vi "ACT_Loop.vi"() -> ()   [LabVIEW 2020, in "Arm_ACT.lvlib"]
uses:
  Arm_ACT.lvlib
  Cluster_CMD_ACT_Data.ctl
  ENUM_ACT_State.ctl
  Type Defs/Talon_FX_Control_Module.ctl
  <vilib>/Rock Robotics/WPI/MotorControl/WPI_MotorControlDeviceRef.ctl
  <vilib>/Rock Robotics/WPI/MotorControl/WPI_MotorControlType.ctl
  <vilib>/Rock Robotics/SystemInterfaces/DIO/FPGA_DIOPWMChannel.ctl
  <vilib>/Rock Robotics/WPI/PWM/WPI_PWMDeadband.ctl
  <vilib>/Rock Robotics/SystemInterfaces/DIO/FPGA_DIOChannel.ctl
  <vilib>/Rock Robotics/WPI/ThirdParty/Phoenix-LabVIEW/Motor Controller/Controls/CTRE_Phoenix_MotorControl_ControlMode.ctl
  ENUM_ACT_Action.ctl
  Utility/Global_STOP.vi
  Global_CMD_ACT_Data In.vi
  <vilib>/Rock Robotics/WPI/ThirdParty/Phoenix-LabVIEW/Motor Controller/Get/CTRE_Phoenix_MotorController_GetLimitSwitchStates.vi
  <vilib>/Rock Robotics/WPI/ThirdParty/Phoenix-LabVIEW/Motor Controller/Get/CTRE_Phoenix_MotorController_GetSelectedSensorData.vi
  Global_ACT_Data Out.vi
panel:
  in  "Arm Offset (Inches)":dbl
  in  "Wrist Offset (Inches)":dbl
  in  "Using Inverse Kinematics?":bool
  in  "arm angle":dbl(slide) scale=0.0..1.0
  out "Input DBL Data":T1
  out "Output DBL Data":dbl
  out "Cycle Time (S)":dbl format="%.3g"
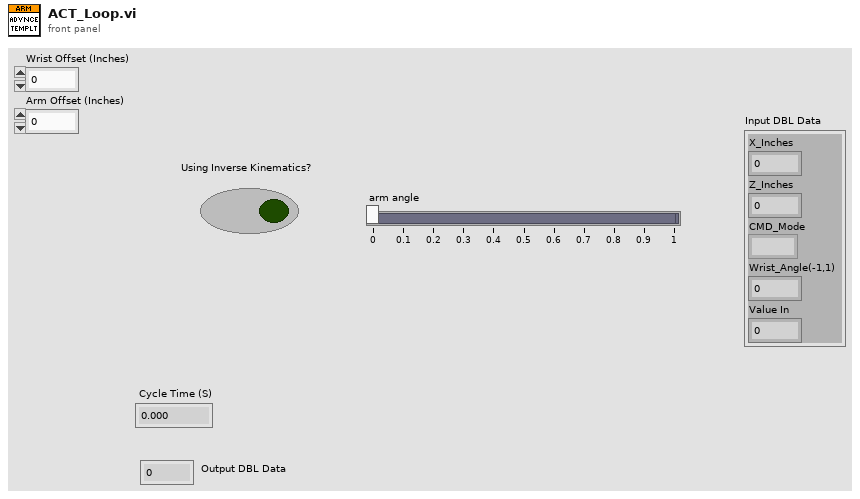
[diagram p1: front panel]
types:
  T1 = typedef "Arm_ACT.lvlib/Cluster_CMD_ACT_Data.ctl" = cluster{"X_Inches":dbl, "Z_Inches":dbl, "CMD_Mode":enum16{""}, "Wrist_Angle(-1,1)":dbl, "Value In":dbl}
  T2 = typedef "Talon_FX_Control_Module.ctl" = cluster{"MotorDevRef":T3, "Control Mode":T8, "Output":dbl}
  T3 = typedef "WPI_MotorControlDeviceRef.ctl" = cluster{"DeviceStatus":errorcluster, "Type":T4, "PWM":cluster{"PWM Channel":T5, "DeadBand":T6}, "CAN":cluster{"Device Number":u8, "SetOutput VI Ref":variant, "GetOutput VI Ref":variant, "Enable VI Ref":variant, "Disable VI Ref":variant, "Data":variant}, "Invert":bool, "DIO PWM":cluster{"PWM \"Enable\" Channel":T5, "DIOChannel":T7, "PWM Rate":dbl}}
  T4 = typedef "WPI_MotorControlType.ctl" = enum16{"PWM", "CAN", "DIO PWM"}
  T5 = typedef "FPGA_DIOPWMChannel.ctl" = enum8{"PWM 0", "PWM 1", "PWM 2", "PWM 3", "PWM 4", "PWM 5", "PWM 6", "PWM 7", "PWM 8", "PWM 9", "PWM MXP 0", "PWM MXP 1", "PWM MXP 2", "PWM MXP 3", "PWM MXP 4", "PWM MXP 5", "PWM MXP 6", "PWM MXP 7", "PWM MXP 8", "PWM MXP 9", "Invalid"}
  T6 = typedef "WPI_PWMDeadband.ctl" = cluster{"Name":string, "maxPositivePwm":i32, "minPositivePwm":i32, "centerPwm":i32, "maxNegativePwm":i32, "minNegativePwm":i32, "angularRange":u16}
  T7 = typedef "FPGA_DIOChannel.ctl" = enum8{"DIO 0", "DIO 1", "DIO 2", "DIO 3", "DIO 4", "DIO 5", "DIO 6", "DIO 7", "DIO 8", "DIO 9", "DIO MXP 0", "DIO MXP 1", "DIO MXP 2", "DIO MXP 3", "DIO MXP 4", "DIO MXP 5", "DIO MXP 6", "DIO MXP 7", "DIO MXP 8", "DIO MXP 9", "DIO MXP 10", "DIO MXP 11", "DIO MXP 12", "DIO MXP 13", "DIO MXP 14", "DIO MXP 15", "SPI Port CS1", "SPI Port CS2", "SPI Port CS3", "SPI Port MISO", "SPI Port MOSI", "Invalid"}
  T8 = typedef "CTRE_Phoenix_MotorControl_ControlMode.ctl" = u16
  T9 = typedef "Arm_ACT.lvlib/ENUM_ACT_State.ctl" = enum16{"Startup", "Set Motors", "Inverse Kinematics Set Motors", "Shutdown"}
  T10 = cluster{"Wrist CM":T2, "Shoulder CM":T2, "Extender CM":T2, "State":T9, "Previous State":T9, "Current Time":timestamp, "Previous Time":timestamp, "Start Time":timestamp, "Target Time (ms)":u32, "Cycle Time(S)":dbl, "ACT Input":T1, "ACT Output DBL":dbl}
  T11 = typedef "Arm_ACT.lvlib/ENUM_ACT_Action.ctl" = enum16{"No Action", "Reset Time", "Reset All", "Zero Motors", "Config Motors", "Set Arm Position", "Set Motors Inverse Kinematics", "Set Wrist Angle"}
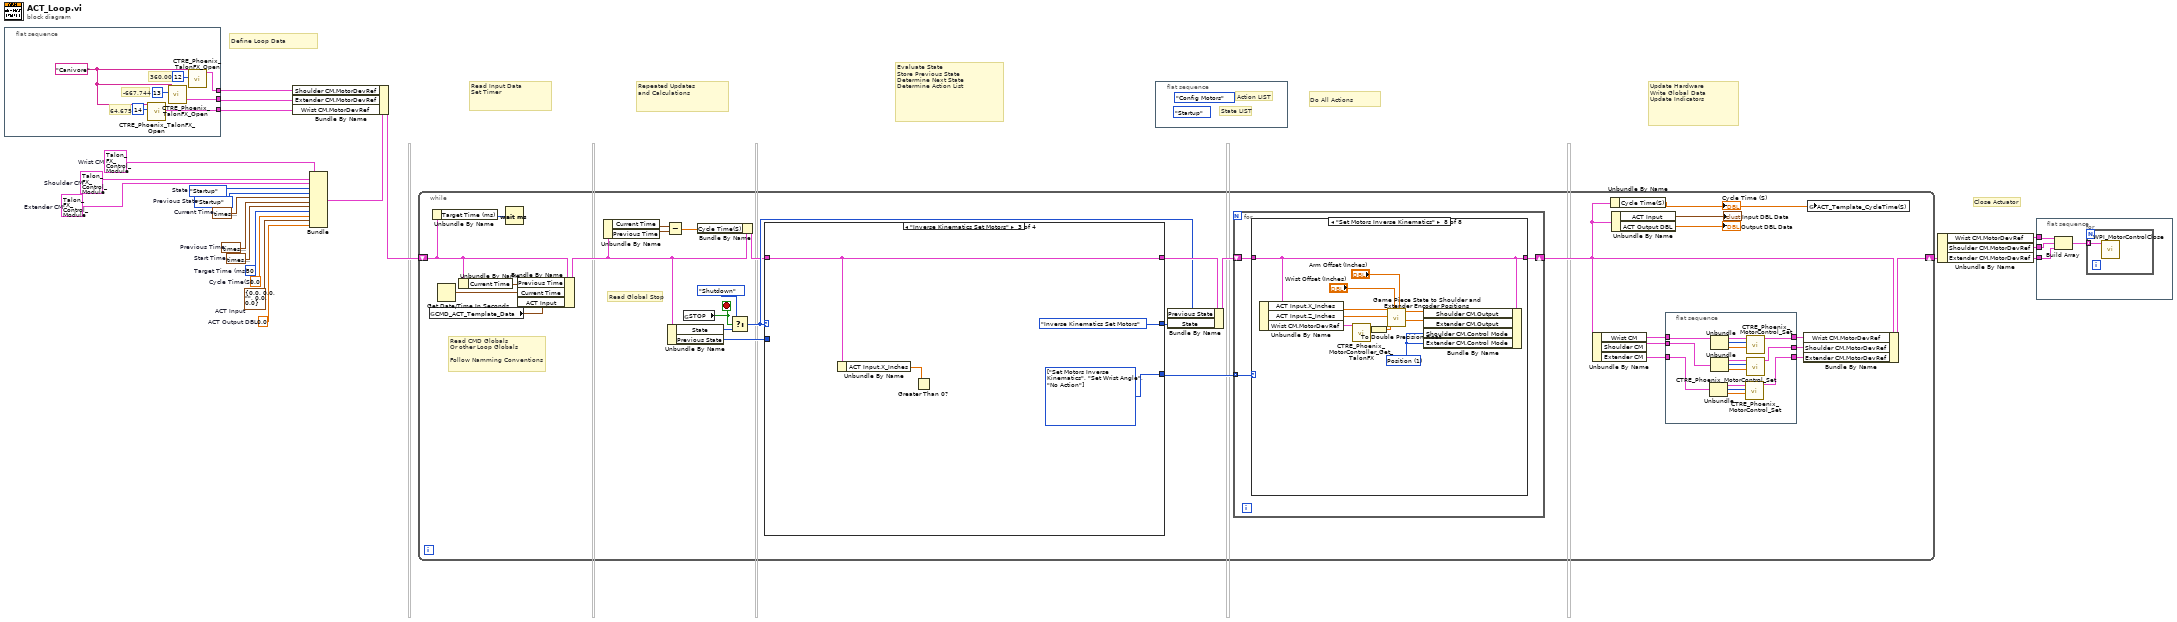
[diagram p0: block diagram]
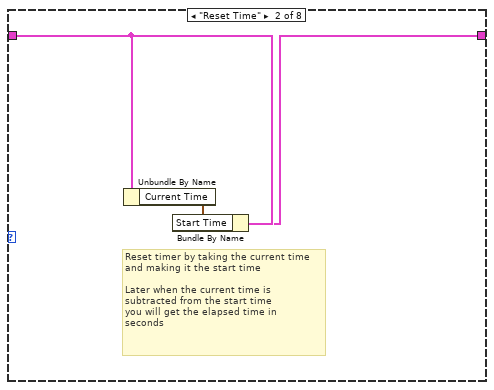
[diagram p3: hidden frame]
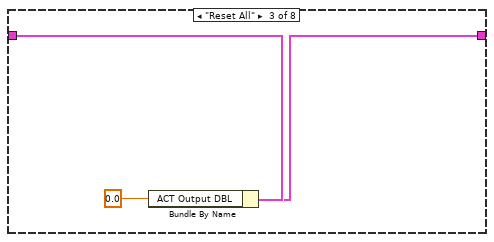
[diagram p4: hidden frame]
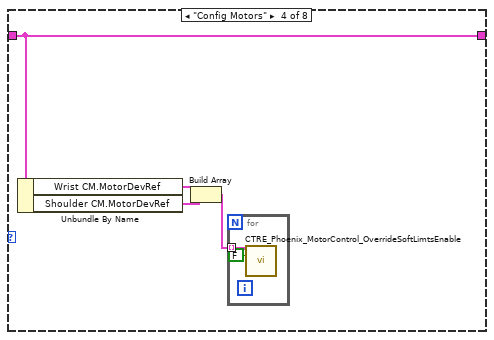
[diagram p5: hidden frame]
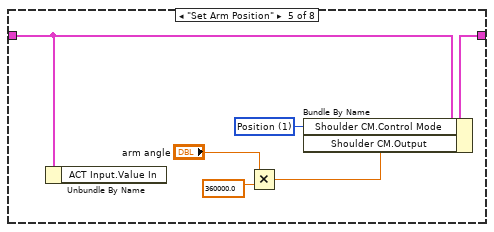
[diagram p6: hidden frame]
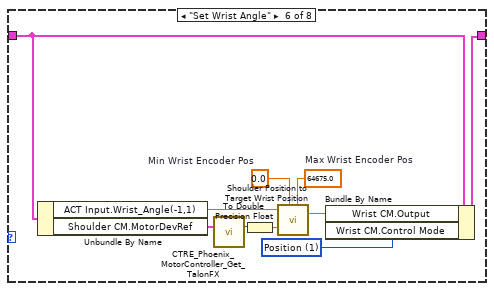
[diagram p7: hidden frame]
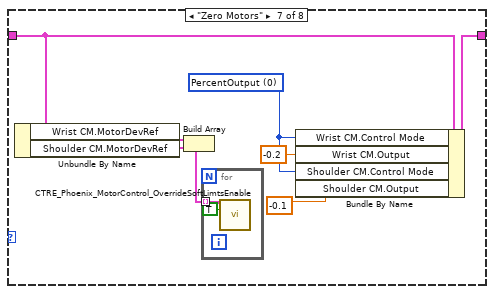
[diagram p8: hidden frame]
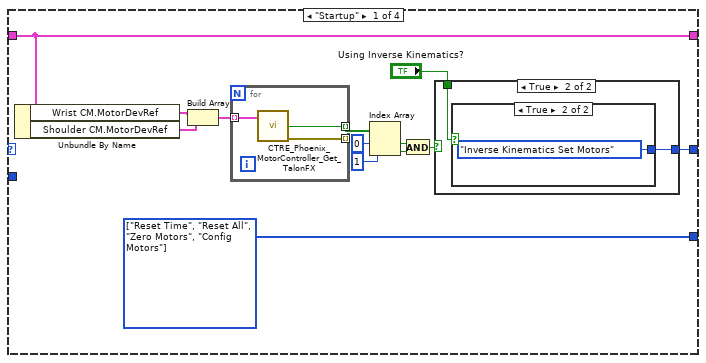
[diagram p9: hidden frame]
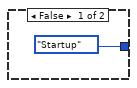
[diagram p10: hidden frame]
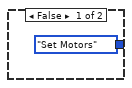
[diagram p11: hidden frame]
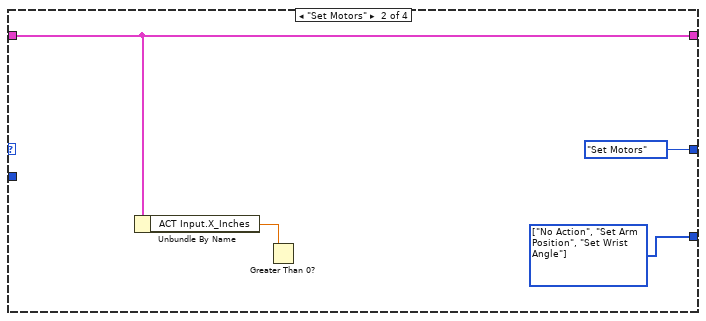
[diagram p12: hidden frame]
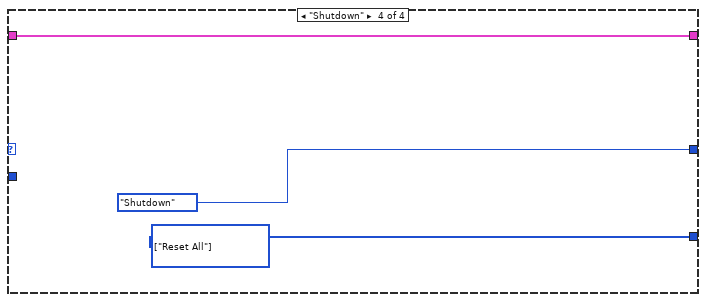
[diagram p13: hidden frame]
diagram:
  w1 = T2 {"MotorDevRef"={"DeviceStatus"={"status"=FALSE, "code"=0, "source"=""}, "Type"=enum."PWM", "PWM"={"PWM Channel"=enum."PWM 1", "DeadBand"={"Name"="", "maxPositivePwm"=0, "minPositivePwm"=0, "centerPwm"=0, "maxNegativePwm"=0, "minNegativePwm"=0, "angularRange"=0}}, "CAN"={"Device Number"=0, "SetOutput VI Ref"=variant(enum8{"Percent VBus", "Current", "Speed", "Position", "Voltage"} enum."Percent VBus"), "GetOutput VI Ref"=variant(refnum<k1> refnum), "Enable VI Ref"=variant(dbl 12.0), "Disable VI Ref"=variant(enum8{"Percent VBus", "Speed", "Position", "Slave", "Unchanged / Invalid", "Voltage Compensation", "Current", "Motion Profile"} enum."Percent VBus"), "Data"=variant}, "Invert"=FALSE, "DIO PWM"={"PWM \"Enable\" Channel"=enum."Invalid", "DIOChannel"=enum."Invalid", "PWM Rate"=0.0}}, "Control Mode"=0, "Output"=0.0}  # Extender CM
  w2 = T2 {"MotorDevRef"={"DeviceStatus"={"status"=FALSE, "code"=0, "source"=""}, "Type"=enum."PWM", "PWM"={"PWM Channel"=enum."PWM 1", "DeadBand"={"Name"="", "maxPositivePwm"=0, "minPositivePwm"=0, "centerPwm"=0, "maxNegativePwm"=0, "minNegativePwm"=0, "angularRange"=0}}, "CAN"={"Device Number"=0, "SetOutput VI Ref"=variant(enum8{"Percent VBus", "Current", "Speed", "Position", "Voltage"} enum."Percent VBus"), "GetOutput VI Ref"=variant(refnum<k1> refnum), "Enable VI Ref"=variant(dbl 12.0), "Disable VI Ref"=variant(enum8{"Percent VBus", "Speed", "Position", "Slave", "Unchanged / Invalid", "Voltage Compensation", "Current", "Motion Profile"} enum."Percent VBus"), "Data"=variant}, "Invert"=FALSE, "DIO PWM"={"PWM \"Enable\" Channel"=enum."Invalid", "DIOChannel"=enum."Invalid", "PWM Rate"=0.0}}, "Control Mode"=0, "Output"=0.0}  # Shoulder CM
  w3 = T2 {"MotorDevRef"={"DeviceStatus"={"status"=FALSE, "code"=0, "source"=""}, "Type"=enum."PWM", "PWM"={"PWM Channel"=enum."PWM 1", "DeadBand"={"Name"="", "maxPositivePwm"=0, "minPositivePwm"=0, "centerPwm"=0, "maxNegativePwm"=0, "minNegativePwm"=0, "angularRange"=0}}, "CAN"={"Device Number"=0, "SetOutput VI Ref"=variant(enum8{"Percent VBus", "Current", "Speed", "Position", "Voltage"} enum."Percent VBus"), "GetOutput VI Ref"=variant(refnum<k1> refnum), "Enable VI Ref"=variant(dbl 12.0), "Disable VI Ref"=variant(enum8{"Percent VBus", "Speed", "Position", "Slave", "Unchanged / Invalid", "Voltage Compensation", "Current", "Motion Profile"} enum."Percent VBus"), "Data"=variant}, "Invert"=FALSE, "DIO PWM"={"PWM \"Enable\" Channel"=enum."Invalid", "DIOChannel"=enum."Invalid", "PWM Rate"=0.0}}, "Control Mode"=0, "Output"=0.0}  # Wrist CM
  w13 = 0.0  # Cycle Time(S)
  w14 = ENUM_ACT_State."Startup"  # Previous State
  w15 = timestamp(0 s since 1904-01-01)  # Previous Time
  w16 = u32 50  # Target Time (ms)
  w17 = 0.0  # ACT Output DBL
  w18 = T1 {"X_Inches"=0.0, "Z_Inches"=0.0, "CMD_Mode"=enum."", "Wrist_Angle(-1,1)"=0.0, "Value In"=0.0}  # ACT Input
  w19 = timestamp(0 s since 1904-01-01)  # Start Time
  w20 = timestamp(0 s since 1904-01-01)  # Current Time
  w21 = ENUM_ACT_State."Startup"  # State
  # "Close Actuator"
  # "Define Loop Data"
  # "Repeated Updates\nand Calculations"
  # "Read Input Data\nSet Timer"
  # "Evaluate State\nStore Previous State\nDetermine Next State\nDetermine Action List"
  # "Do All Actions"
  # "Update Hardware\nWrite Global Data\nUpdate Indicators"
  n1 = flat-sequence {
    tunnel: [w27] -> w8
    tunnel: [w25] -> w7
    tunnel: [w23] -> w6
    frame #0 {
      w22 = "Canivore" ("CAN Bus")
      # "360,000"
      # "-667,744"
      # "64,675"
      n2 = call <vilib>:"CTRE_Phoenix_TalonFX_Open.vi"("Device Number"=u8 14, "CAN Bus"=w22) -> ("PhoenixMotorControlDevRef"=w27:T3)  [unwired: 8 in, 1 out]
      n3 = call <vilib>:"CTRE_Phoenix_TalonFX_Open.vi"("Device Number"=u8 13, "CAN Bus"=w22) -> ("PhoenixMotorControlDevRef"=w25:T3)  [unwired: 8 in, 1 out]
      n4 = call <vilib>:"CTRE_Phoenix_TalonFX_Open.vi"("Device Number"=u8 12, "CAN Bus"=w22) -> ("PhoenixMotorControlDevRef"=w23:T3)  [unwired: 8 in, 1 out]
    }
  }
  n5 = Bundle("Wrist CM"=w3, "Shoulder CM"=w2, "Extender CM"=w1, "State"=w21, "Previous State"=w14, "Current Time"=w20, "Previous Time"=w15, "Start Time"=w19, "Target Time (ms)"=w16, "Cycle Time(S)"=w13, "ACT Input"=w18, "ACT Output DBL"=w17) -> (w10:T10)  [unwired: 1 in]
  n6 = Bundle By Name(cluster=w10, "Shoulder CM.MotorDevRef"=w6, "Extender CM.MotorDevRef"=w7, "Wrist CM.MotorDevRef"=w8) -> (w9:T10)
  n7 = while {
    shift-right: [w37] -> w11
    shift-left: w9 -> [w33]
    stop <- w54 stop-if-true
    # "Read CMD Globals\nOr other Loop Globals\n\nFollow Namming Conventions"
    # "Read Global Stop"
    n8 = global read "Global_CMD_ACT_Data In.vi" "CMD_ACT_Template_Data"() -> (w39:T1)
    n9 = Unbundle By Name(w33) -> ("Target Time (ms)"=w51:u32)
    n10 = Get Date/Time In Seconds() -> (seconds since 1Jan1904=w58:timestamp)
    n11 = Unbundle By Name(w33) -> ("Current Time"=w50:timestamp)
    n12 = Wait (ms)(milliseconds to wait=w51) -> ()  [unwired: 1 out]
    n13 = Bundle By Name(cluster=w33, "Previous Time"=w50, "Current Time"=w58, "ACT Input"=w39) -> (w44:T10)
    n14 = Unbundle By Name(w44) -> ("Current Time"=w45:timestamp, "Previous Time"=w46:timestamp)
    n15 = Subtract(x=w45, y=w46) -> (x-y=w42:dbl)
    n16 = Unbundle By Name(w44) -> ("State"=w52:T9, "Previous State"=w49:T9)
    n17 = global read "Global_STOP.vi" "STOP"() -> (w54:bool)
    n18 = Bundle By Name(cluster=w44, "Cycle Time(S)"=w42) -> (w43:T10)
    n19 = Select(t=ENUM_ACT_State."Shutdown" ("State"), s=w54, f=w52) -> (s? t:f=w47:T9)
    n20 = case shown="\"Inverse Kinematics Set Motors\"" w47 {
      tunnel: w43 -> [w137 w149 w153 w158]
      tunnel: [w137 w149 w153 w158] -> w56
      tunnel: [w138 ENUM_ACT_State."Set Motors" ("State") ENUM_ACT_State."Inverse Kinematics Set Motors" ("State") ENUM_ACT_State."Shutdown" ("State")] -> w55
      tunnel: [w139 w148 w152 w156] -> w41
      tunnel: w49 -> [_ _ _ _]
      frame "Startup" {
        w139 = T11[] [enum."Reset Time", enum."Reset All", enum."Zero Motors", enum."Config Motors"] items=["No Action", "Reset Time", "Reset All", "Zero Motors", "Config Motors", "Set Arm Position", "Set Motors Inverse Kinematics", "Set Wrist Angle"] ("Actions")
        n21 = Unbundle By Name(w137) -> ("Wrist CM.MotorDevRef"=w136:T3, "Shoulder CM.MotorDevRef"=w128:T3)
        n22 = Build Array(w136, w128) -> (w134:T3[])
        n23 = for {
          tunnel: w134 -> [w142] mode=indexing
          tunnel: [w141] -> w133 mode=indexing
          tunnel: [w140] -> _ mode=indexing
          n24 = call-poly <vilib>:"CTRE_Phoenix_MotorController_Get_TalonFX.vi"("PhoenixMotorControlDevRef"=w142) -> ("Reverse Limit Closed?"=w141:bool, "error out"=w140:errorcluster)  [unwired: 11 in, 2 out]
        }
        n25 = Index Array(array=w133, index #1=0 ("index"), index #2=1 ("index")) -> (element #1=w130:bool, element #2=w129:bool)
        n26 = And(x=w130, y=w129) -> (x .and. y?=w135:bool)
        n27 = case shown="True" w135 {
          tunnel: [ENUM_ACT_State."Startup" ("State") w145] -> w138
          tunnel: "Using Inverse Kinematics?" -> [_ w144]
          frame False {
          }
          frame True {
            n28 = case shown="True" w144 {
              tunnel: [ENUM_ACT_State."Set Motors" ("State") ENUM_ACT_State."Inverse Kinematics Set Motors" ("State")] -> w145
              frame False {
              }
              frame True {
              }
            }
          }
        }
      }
      frame "Set Motors" {
        w148 = T11[] [enum."No Action", enum."Set Arm Position", enum."Set Wrist Angle"] items=["No Action", "Reset Time", "Reset All", "Zero Motors", "Config Motors", "Set Arm Position", "Set Motors Inverse Kinematics", "Set Wrist Angle"] ("Actions")
        n29 = Unbundle By Name(w149) -> ("ACT Input.X_Inches"=w151:dbl)
        n30 = Greater Than 0?(x=w151) -> ()  [unwired: 1 out]
      }
      frame "Inverse Kinematics Set Motors" {
        w152 = T11[] [enum."Set Motors Inverse Kinematics", enum."Set Wrist Angle", enum."No Action"] items=["No Action", "Reset Time", "Reset All", "Zero Motors", "Config Motors", "Set Arm Position", "Set Motors Inverse Kinematics", "Set Wrist Angle"] ("Actions")
        n31 = Unbundle By Name(w153) -> ("ACT Input.X_Inches"=w155:dbl)
        n32 = Greater Than 0?(x=w155) -> ()  [unwired: 1 out]
      }
      frame "Shutdown" {
        w156 = T11[] [enum."Reset All"] items=["No Action", "Reset Time", "Reset All", "Zero Motors", "Config Motors", "Set Arm Position", "Set Motors Inverse Kinematics", "Set Wrist Angle"] ("Actions")
      }
    }
    n33 = Bundle By Name(cluster=w56, "Previous State"=w47, "State"=w55) -> (w57:T10)
    n34 = for {
      tunnel: w41 -> [w76] mode=indexing
      shift-right: [w75] -> w38
      shift-left: w57 -> [w74]
      n35 = case shown="\"Set Motors Inverse Kinematics\"" w76 {
        tunnel: w74 -> [w77 w80 w83 w85 w95 w99 w110 w119]
        tunnel: [w77 w79 w82 w85 w94 w98 w109 w119] -> w75
        frame "No Action" {
        }
        frame "Reset Time" {
          # "Reset timer by taking the current time\nand making it the start time\n\nLater when the current time is \nsubtracted from the start time\nyou will get the elapsed time in \nseconds"
          n36 = Unbundle By Name(w80) -> ("Current Time"=w78:timestamp)
          n37 = Bundle By Name(cluster=w80, "Start Time"=w78) -> (w79:T10)
        }
        frame "Reset All" {
          n38 = Bundle By Name(cluster=w83, "ACT Output DBL"=0.0 ("FG Write Value")) -> (w82:T10)
        }
        frame "Config Motors" {
          n39 = Unbundle By Name(w85) -> ("Wrist CM.MotorDevRef"=w87:T3, "Shoulder CM.MotorDevRef"=w86:T3)
          n40 = Build Array(w87, w86) -> (w84:T3[])
          n41 = for {
            tunnel: w84 -> [w89] mode=indexing
            n42 = call <vilib>:"CTRE_Phoenix_MotorControl_OverrideSoftLimtsEnable.vi"("PhoenixMotorControlDevRef"=w89, "Override Soft Limit Enable?"=FALSE) -> ()  [unwired: 12 in, 2 out]
          }
        }
        frame "Set Arm Position" {
          w93 = T8 1 items=["PercentOutput"=0, "Position"=1, "Velocity"=2, "Current"=3, "Follower"=5, "MotionProfile"=6, "MotionMagic"=7, "MotionProfileArc"=10, "Disabled"=15] ("Shoulder CM.Control Mode")
          n43 = Unbundle By Name(w95) -> ()  [unwired: 1 out]
          n44 = Multiply(x="arm angle", y=360000.0) -> (x*y=w91:dbl)
          n45 = Bundle By Name(cluster=w95, "Shoulder CM.Control Mode"=w93, "Shoulder CM.Output"=w91) -> (w94:T10)
        }
        frame "Set Wrist Angle" {
          w97 = T8 1 items=["PercentOutput"=0, "Position"=1, "Velocity"=2, "Current"=3, "Follower"=5, "MotionProfile"=6, "MotionMagic"=7, "MotionProfileArc"=10, "Disabled"=15] ("Wrist Control Mode")
          w100 = 64675.0  # Max Wrist Encoder Pos
          w101 = 0.0  # Min Wrist Encoder Pos
          n46 = Unbundle By Name(w99) -> ("ACT Input.Wrist_Angle(-1,1)"=w102:dbl, "Shoulder CM.MotorDevRef"=w105:T3)
          n47 = call-poly <vilib>:"CTRE_Phoenix_MotorController_Get_TalonFX.vi"("PhoenixMotorControlDevRef"=w105) -> ("Position (Raw Sensor Units)"=w104:i32)  [unwired: 11 in, 3 out]
          n48 = To Double Precision Float(number=w104) -> (double precision float=w103:dbl)
          n49 = call "Shoulder Position to Target Wrist Position.vi"("Wrist Encoder Pos at 90 degrees"=w100, "Min Wrist Encoder Pos"=w101, "Shoulder Enc Position"=w103, "Wanted Wrist Angle (-1,1)"=w102) -> ("Target Wrist Enc Position"=w96:dbl)  [unwired: 7 in]
          n50 = Bundle By Name(cluster=w99, "Wrist CM.Output"=w96, "Wrist CM.Control Mode"=w97) -> (w98:T10)
        }
        frame "Zero Motors" {
          w108 = T8 0 items=["PercentOutput"=0, "Position"=1, "Velocity"=2, "Current"=3, "Follower"=5, "MotionProfile"=6, "MotionMagic"=7, "MotionProfileArc"=10, "Disabled"=15] ("Wrist CM.Control Mode")
          n51 = Unbundle By Name(w110) -> ("Wrist CM.MotorDevRef"=w113:T3, "Shoulder CM.MotorDevRef"=w112:T3)
          n52 = Build Array(w113, w112) -> (w111:T3[])
          n53 = for {
            tunnel: w111 -> [w115] mode=indexing
            n54 = call <vilib>:"CTRE_Phoenix_MotorControl_OverrideSoftLimtsEnable.vi"("PhoenixMotorControlDevRef"=w115, "Override Soft Limit Enable?"=TRUE) -> ()  [unwired: 12 in, 2 out]
          }
          n55 = Bundle By Name(cluster=w110, "Wrist CM.Control Mode"=w108, "Wrist CM.Output"=-0.2, "Shoulder CM.Control Mode"=w108, "Shoulder CM.Output"=-0.1) -> (w109:T10)
        }
        frame "Set Motors Inverse Kinematics" {
          w116 = T8 1 items=["PercentOutput"=0, "Position"=1, "Velocity"=2, "Current"=3, "Follower"=5, "MotionProfile"=6, "MotionMagic"=7, "MotionProfileArc"=10, "Disabled"=15] ("Extender CM.Control Mode")
          n56 = Unbundle By Name(w119) -> ("ACT Input.X_Inches"=w126:dbl, "ACT Input.Z_Inches"=w125:dbl, "Wrist CM.MotorDevRef"=w124:T3)
          n57 = call-poly <vilib>:"CTRE_Phoenix_MotorController_Get_TalonFX.vi"("PhoenixMotorControlDevRef"=w124) -> ("Position (Raw Sensor Units)"=w123:i32)  [unwired: 11 in, 3 out]
          n58 = To Double Precision Float(number=w123) -> (double precision float=w122:dbl)
          n59 = call "Game Piece State to Shoulder and Extender Encoder Positions.vi"("Arm Offset (Inches)"="Arm Offset (Inches)", "Wrist Offset (Inches)"="Wrist Offset (Inches)", "Wrist Enc Position"=w122, "Z (Inches)"=w125, "X (Inches)"=w126) -> ("Target Extender Enc Pos"=w117:dbl, "Target Shoulder Enc Pos"=w118:dbl)  [unwired: 5 in]
          n60 = Bundle By Name(cluster=w119, "Shoulder CM.Output"=w118, "Extender CM.Output"=w117, "Shoulder CM.Control Mode"=w116, "Extender CM.Control Mode"=w116) -> ()  [unwired: 1 out]
        }
      }
    }
    n61 = Unbundle By Name(w38) -> ("Wrist CM"=w34:T2, "Shoulder CM"=w32:T2, "Extender CM"=w29:T2)
    n62 = Unbundle By Name(w38) -> ("Cycle Time(S)"=w36:dbl)
    "Cycle Time (S)" <- w36
    n63 = Unbundle By Name(w38) -> ("ACT Input"=→"Input DBL Data":T1, "ACT Output DBL"=→"Output DBL Data":dbl)
    n64 = flat-sequence {
      tunnel: [w73] -> w35
      tunnel: w34 -> [w69]
      tunnel: w32 -> [w65]
      tunnel: [w64] -> w31
      tunnel: [w61] -> w30
      tunnel: w29 -> [w60]
      frame #0 {
        n65 = Unbundle(w60) -> ("MotorDevRef"=w59:T3, "Control Mode"=w63:T8, "Output"=w62:dbl)
        n66 = Unbundle(w69) -> ("MotorDevRef"=w72:T3, "Control Mode"=w71:T8, "Output"=w70:dbl)
        n67 = Unbundle(w65) -> ("MotorDevRef"=w68:T3, "Control Mode"=w67:T8, "Output"=w66:dbl)
        n68 = call <vilib>:"CTRE_Phoenix_MotorControl_Set.vi"("Output"=w62, "Control Mode"=w63, "PhoenixMotorControlDevRef"=w59) -> ("PhoenixMotorControlDevRef"=w61:T3)  [unwired: 7 in, 1 out]
        n69 = call <vilib>:"CTRE_Phoenix_MotorControl_Set.vi"("Output"=w70, "Control Mode"=w71, "PhoenixMotorControlDevRef"=w72) -> ("PhoenixMotorControlDevRef"=w73:T3)  [unwired: 7 in, 1 out]
        n70 = call <vilib>:"CTRE_Phoenix_MotorControl_Set.vi"("Output"=w66, "Control Mode"=w67, "PhoenixMotorControlDevRef"=w68) -> ("PhoenixMotorControlDevRef"=w64:T3)  [unwired: 7 in, 1 out]
      }
    }
    n71 = Bundle By Name(cluster=w38, "Wrist CM.MotorDevRef"=w35, "Shoulder CM.MotorDevRef"=w31, "Extender CM.MotorDevRef"=w30) -> (w37:T10)
    n72 = global write "Global_ACT_Data Out.vi" "ACT_Template_CycleTime(S)"(w36) -> ()
  }
  n73 = flat-sequence {
    frame #0 {
      (unwired) ENUM_ACT_State."Startup" ("State")
      (unwired) ENUM_ACT_Action."Config Motors" ("Action")
      # "State LIST"
      # "Action LIST"
    }
  }
  n74 = Unbundle By Name(w11) -> ("Wrist CM.MotorDevRef"=w4:T3, "Shoulder CM.MotorDevRef"=w5:T3, "Extender CM.MotorDevRef"=w12:T3)
  n75 = flat-sequence {
    tunnel: w12 -> [w160]
    tunnel: w5 -> [w161]
    tunnel: w4 -> [w162]
    frame #0 {
      n76 = Build Array(w162, w161, w160) -> (w159:T3[])
      n77 = for {
        tunnel: w159 -> [w163] mode=indexing
        n78 = call <vilib>:"WPI_MotorControlClose.vi"("MotorControlDevRef"=w163) -> ()  [unwired: 10 in, 1 out]
      }
    }
  }
